vi "Parse Error XML.vi"(9 "Code Tag Value":string, 10 "Error XML":string, 11 "AWS Core":refnum<class "Topic.lvclass">) -> (1 "Error Description Override":string, 2 "Error Code":i32, 3 "Warning":bool)   [LabVIEW 2015, in "NI_AWS_SNS.lvlib" / "Topic.lvclass"]
uses:
  Topic.lvclass
  Core/ARN/ARN.lvclass
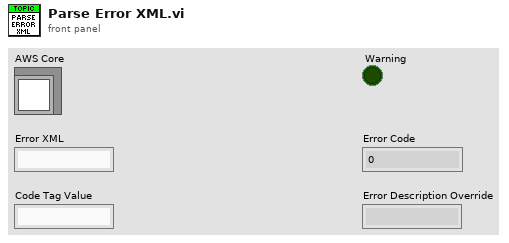
[diagram p1: front panel]
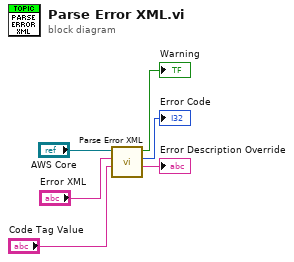
[diagram p0: block diagram]
diagram:
  n1 = call-parent "Parse Error XML.vi"("Code Tag Value"="Code Tag Value", "Error XML"="Error XML", "AWS Core"="AWS Core") -> ("Error Description Override"=→"Error Description Override":string, "Error Code"=→"Error Code":i32, "Warning"=→"Warning":bool)  [unwired: 6 in]
